vi "CreateRGB_Imgs.vi"() -> (0 "Blue":T1, 1 "Green":T1, 2 "Red":T1, 3 "RGB Cluster":cluster{"Red":T1, "Green":T1, "Blue":T1})   [LabVIEW 2013]
uses:
  <vilib>/vision/Image Controls.llb/IMAQ Image.ctl
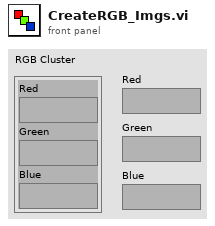
[diagram p1: front panel]
types:
  T1 = typedef "IMAQ Image.ctl" = refnum<image>
  T2 = typedef "Image Type" = u32
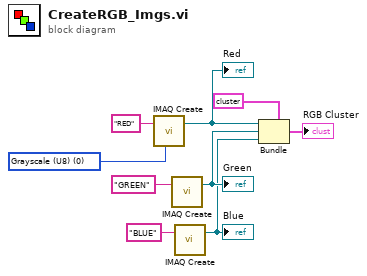
[diagram p0: block diagram]
diagram:
  w8 = T2 0 items=["Grayscale (U8)", "Grayscale (I16)", "Grayscale (SGL)", "Complex (CSG)", "RGB (U32)", "HSL (U32)", "RGB (U64)", "Grayscale (U16)"] ("Image Type")
  n1 = call "IMAQ Create"("Image Name"="RED", "Image Type"=w8) -> ("New Image"=w6:T1)  [unwired: 3 in, 1 out]
  "Red" <- w6
  n2 = call "IMAQ Create"("Image Name"="GREEN") -> ("New Image"=w5:T1)  [unwired: 4 in, 1 out]
  "Green" <- w5
  n3 = call "IMAQ Create"("Image Name"="BLUE") -> ("New Image"=w4:T1)  [unwired: 4 in, 1 out]
  "Blue" <- w4
  n4 = Bundle(cluster=cluster{"Red":T1, "Green":T1, "Blue":T1} {"Red"=refnum, "Green"=refnum, "Blue"=refnum}, "Red"=w6, "Green"=w5, "Blue"=w4) -> (→"RGB Cluster":cluster{"Red":T1, "Green":T1, "Blue":T1})
